vi "Get Display String.vi"(11 "Str Contains in":refnum<class "Str Contains.lvclass">) -> (2 "Display String":string)   [LabVIEW 2018, in "Str Contains.lvclass"]
uses:
  Str Contains.lvclass
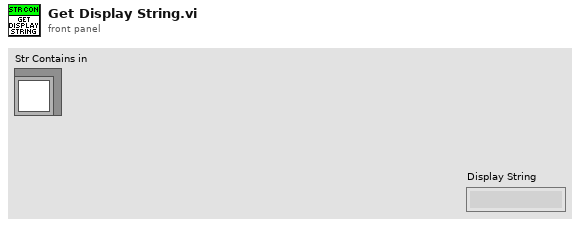
[diagram p1: front panel]
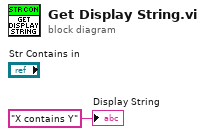
[diagram p0: block diagram]
diagram:
  "Display String" <- "X contains Y" ("Display String")
